vi "Order of Polynomial.vi"   [LabVIEW 2020, in "NI_AALPro.lvlib"]
doc: "Finds the order, or polynomial degree, of polynomial <B>P(x)</B>. Wire data to the <B>P(x)</B> input to determine the polymorphic instance to use or manually select the instance."
uses:
  NI_AALPro.lvlib
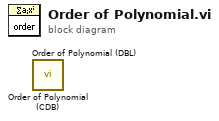
[diagram p0: block diagram]
diagram:
  n1 = call "Order of Polynomial (CDB).vi"() -> ()  [unwired: 10 in, 2 out]
  n2 = call "Order of Polynomial (DBL).vi"() -> ()  [unwired: 10 in, 2 out]
